vi "ServoCOMPLEX.vi"() -> ()   [LabVIEW 2016]
panel:
  out "Power on sample":dbl
  in  "Ring":u16(ring) items=["xx mW (ND0.04)", "xx mW (ND0.5)", "xx mW (ND1)", "xx mW (ND1.5)"]
  in  "Power Before Pinhole":dbl
  out "Sample Plane Init":dbl
  out "Before Pinhole Init":dbl
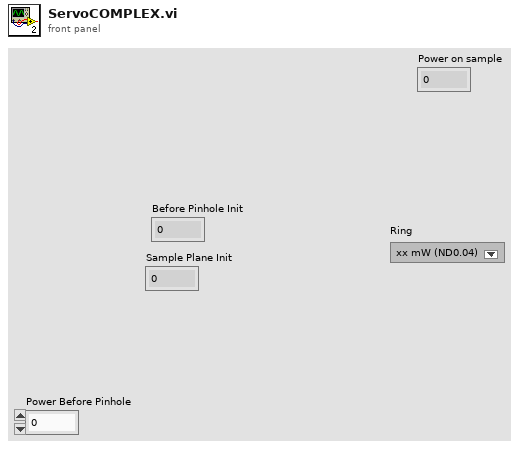
[diagram p1: front panel]
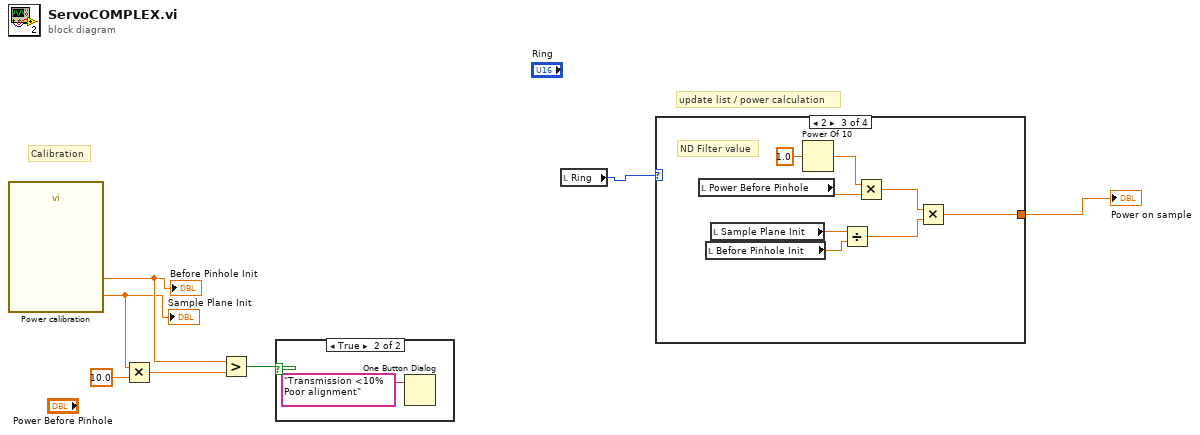
[diagram p0: block diagram]
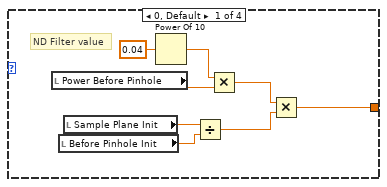
[diagram p2: hidden frame]
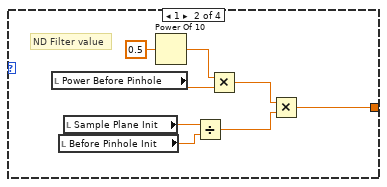
[diagram p3: hidden frame]
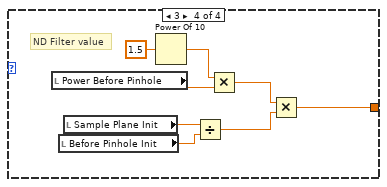
[diagram p4: hidden frame]
diagram:
  # "update list / power calculation"
  # "Calibration"
  n1 = call "Power calibration"() -> ("Sample Power"=w5:dbl, "Input Power"=w7:dbl)  [unwired: 16 in, 2 out]
  "Before Pinhole Init" <- w7
  "Sample Plane Init" <- w5
  n2 = Multiply(x=w5, y=10.0) -> (x*y=w6:dbl)
  n3 = Greater?(x=w7, y=w6) -> (0:w3:bool)
  n4 = case shown="True" w3 {
    frame False {
    }
    frame True {
      n5 = One Button Dialog(message="Transmission <10% Poor alignment") -> ()  [unwired: 1 in, 1 out]
    }
  }
  n6 = local read "Ring"() -> (w1:u16)
  n7 = case shown="2" w1 {
    tunnel: [w9 w17 w25 w33] -> w2
    frame 0, Default {
      # "ND Filter value"
      n8 = local read "Power Before Pinhole"() -> (w16:dbl)
      n9 = local read "Before Pinhole Init"() -> (w12:dbl)
      n10 = local read "Sample Plane Init"() -> (w13:dbl)
      n11 = Power Of 10(x=0.04) -> (10^x=w14:dbl)
      n12 = Divide(x=w13, y=w12) -> (x/y=w10:dbl)
      n13 = Multiply(x=w14, y=w16) -> (x*y=w11:dbl)
      n14 = Multiply(x=w11, y=w10) -> (x*y=w9:dbl)
    }
    frame 1 {
      # "ND Filter value"
      n15 = local read "Power Before Pinhole"() -> (w24:dbl)
      n16 = local read "Before Pinhole Init"() -> (w20:dbl)
      n17 = local read "Sample Plane Init"() -> (w21:dbl)
      n18 = Power Of 10(x=0.5) -> (10^x=w22:dbl)
      n19 = Divide(x=w21, y=w20) -> (x/y=w18:dbl)
      n20 = Multiply(x=w22, y=w24) -> (x*y=w19:dbl)
      n21 = Multiply(x=w19, y=w18) -> (x*y=w17:dbl)
    }
    frame 2 {
      # "ND Filter value"
      n22 = local read "Power Before Pinhole"() -> (w32:dbl)
      n23 = local read "Before Pinhole Init"() -> (w28:dbl)
      n24 = local read "Sample Plane Init"() -> (w29:dbl)
      n25 = Power Of 10(x=1.0) -> (10^x=w30:dbl)
      n26 = Divide(x=w29, y=w28) -> (x/y=w26:dbl)
      n27 = Multiply(x=w30, y=w32) -> (x*y=w27:dbl)
      n28 = Multiply(x=w27, y=w26) -> (x*y=w25:dbl)
    }
    frame 3 {
      # "ND Filter value"
      n29 = local read "Power Before Pinhole"() -> (w40:dbl)
      n30 = local read "Before Pinhole Init"() -> (w36:dbl)
      n31 = local read "Sample Plane Init"() -> (w37:dbl)
      n32 = Power Of 10(x=1.5) -> (10^x=w38:dbl)
      n33 = Divide(x=w37, y=w36) -> (x/y=w34:dbl)
      n34 = Multiply(x=w38, y=w40) -> (x*y=w35:dbl)
      n35 = Multiply(x=w35, y=w34) -> (x*y=w33:dbl)
    }
  }
  "Power on sample" <- w2
